vi "Flush.vi"(8 "error in (no error)":errorcluster, 11 "UPNCalculator in":refnum<class "UPNCalculator.lvclass">) -> (0 "error out":errorcluster, 3 "UPNCalculator out":refnum<class "UPNCalculator.lvclass">)   [LabVIEW 2016, in "UPNCalculator Actor.lvlib" / "UPNCalculator.lvclass"]
doc: "Flush content from stack."
uses:
  UPNCalculator.lvclass
  UPNCalculator.lvclass/UPNCalculator.ctl
  Stack/Stack.lvclass
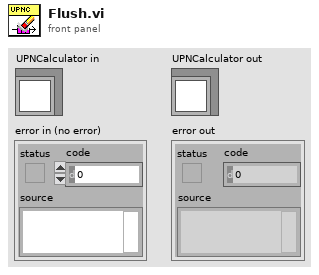
[diagram p1: front panel]
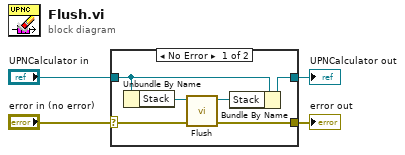
[diagram p0: block diagram]
diagram:
  n1 = case shown="No Error" "error in (no error)" {
    selector: "error in (no error)" -> [w9 w12]
    tunnel: [w8 w12] -> w3
    tunnel: [w6 w11] -> w1
    tunnel: "UPNCalculator in" -> [w7 w11]
    frame No Error {
      n2 = Unbundle By Name(w7) -> ("Stack"=w10:refnum<class "Stack.lvclass">)
      n3 = call "Flush.vi"("error in (no error)"=w9, "Stack in"=w10) -> ("error out"=w8:errorcluster, "Stack out"=w5:refnum<class "Stack.lvclass">)  [unwired: 8 in]
      n4 = Bundle By Name(cluster=w7, "Stack"=w5) -> (w6:refnum<class "UPNCalculator.lvclass">)
    }
    frame Error {
    }
  }
  "error out" <- w3
  "UPNCalculator out" <- w1
